vi "Bundle ISD time domain files.vi"(11 "path":path) -> ()   [LabVIEW 2020]
uses:
  <vilib>/Utility/file.llb/Read Delimited Spreadsheet (DBL).vi
  <vilib>/Utility/file.llb/Write Delimited Spreadsheet (string).vi
  <vilib>/Utility/file.llb/Write Delimited Spreadsheet (DBL).vi
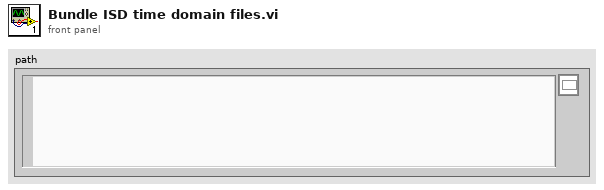
[diagram p1: front panel]
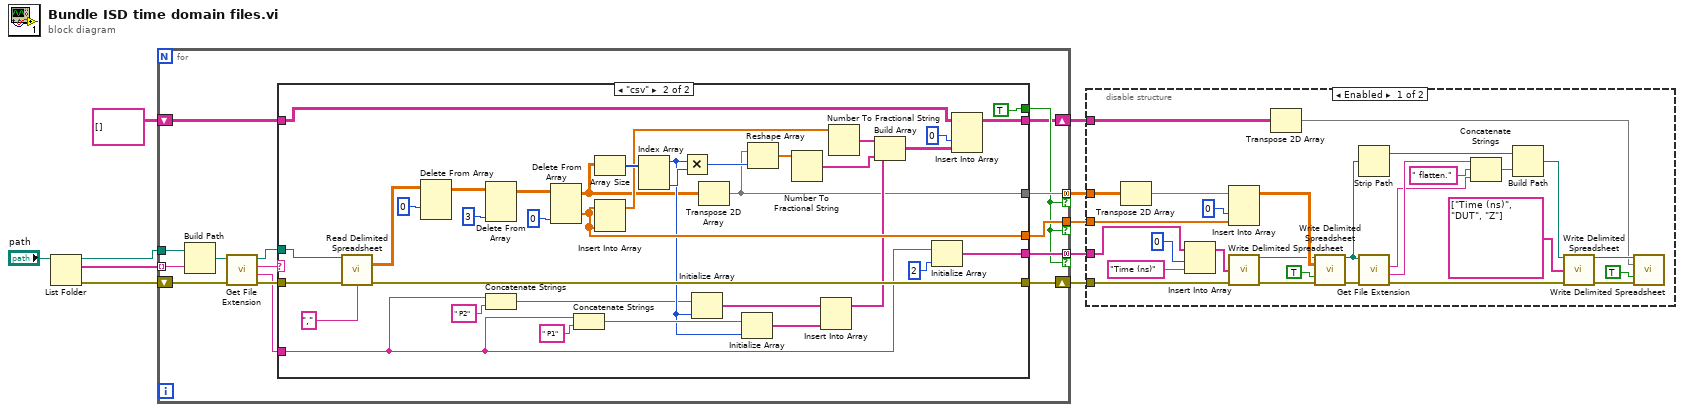
[diagram p0: block diagram]
diagram:
  n1 = List Folder(path="path") -> (path out=w10:path, filenames=w9:string[], error out=w8:errorcluster)  [unwired: 3 in, 1 out]
  n2 = for {
    tunnel: w10 -> [w24]
    tunnel: w9 -> [w23] mode=indexing
    shift-right: [w19] -> w1
    shift-left: w8 -> [w21]
    tunnel: [w17] -> w6 mode=concatenating if=w13
    tunnel: [w16] -> w5 if=w13
    tunnel: [w14] -> w4 mode=concatenating if=w13
    shift-right: [w12] -> w2
    shift-left: string[][] [] -> [w11]
    n3 = Build Path(base path=w24, name or relative path=w23) -> (appended path=w22:path)
    n4 = call <vilib>:"Get File Extension.vi"("error in (no error)"=w21, "file"=w22) -> ("error out"=w20:errorcluster, "filename without extension"=w15:string, "lowercase file extension"=w25:string, "dup file"=w18:path)  [unwired: 5 in, 1 out]
    n5 = case shown="\"csv\"" w25 {
      tunnel: w20 -> [w27 w63]
      tunnel: [w27 w61] -> w19
      tunnel: w18 -> [_ w60]
      tunnel: [_ w28] -> w17
      tunnel: [_ TRUE] -> w13
      tunnel: [_ w40] -> w16
      tunnel: w15 -> [_ w36]
      tunnel: [_ w53] -> w14
      tunnel: [w26 w51] -> w12
      tunnel: w11 -> [w26 w52]
      frame "False", Default {
      }
      frame "csv" {
        n6 = call-poly <vilib>:"Read Delimited Spreadsheet.vi"("file path (dialog if empty)"=w60, "error in (no error)"=w63, "delimiter (\\t)"="," ("delimiter (\\t)")) -> ("all rows"=w57:dbl[][], "error out"=w61:errorcluster)  [unwired: 7 in, 4 out]
        n7 = Delete From Array(array=w57, index (row)=0 ("index")) -> (array with subset deleted=w58:dbl[][])  [unwired: 2 in, 1 out]
        n8 = Delete From Array(array=w58, index (col)=3 ("disabled index (col)")) -> (array with subset deleted=w49:dbl[][])  [unwired: 2 in, 1 out]
        n9 = Concatenate Strings(w36, " P2" ("string")) -> (w30:string)
        n10 = Delete From Array(array=w49, index (col)=0 ("disabled index (col)")) -> (deleted portion=w40:dbl[], array with subset deleted=w29:dbl[][])  [unwired: 2 in]
        n11 = Concatenate Strings(w36, " P1" ("string")) -> (w35:string)
        n12 = Array Size(array=w29) -> (size(s)=w48:i32[])
        n13 = Insert Into Array(array=w40, new element=w40) -> (w39:dbl[])  [unwired: 1 in]
        n14 = Index Array(array=w48) -> (element #1=w34:i32, element #2=w47:i32)  [unwired: 2 in]
        n15 = Multiply(x=w34, y=w47) -> (x*y=w46:i32)
        n16 = Initialize Array(w30, w34) -> (w33:string[])
        n17 = Transpose 2D Array(2D array=w29) -> (transposed array=w28:dbl[][])
        n18 = Initialize Array(w35, w34) -> (w32:string[])
        n19 = Reshape Array(w28, w46) -> (w43:dbl[])
        n20 = Number To Fractional String(number=w43) -> (F-format string=w42:string[])  [unwired: 3 in]
        n21 = Insert Into Array(array=w33, new element=w32) -> (w31:string[])  [unwired: 1 in]
        n22 = Number To Fractional String(number=w39) -> (F-format string=w41:string[])  [unwired: 3 in]
        n23 = Build Array(w41, w31, w42) -> (w45:string[][])
        n24 = Initialize Array(w36, 2 ("dimension size")) -> (w53:string[])
        n25 = Insert Into Array(array=w52, index (col)=0 ("disabled index (col)"), new element=w45) -> (w51:string[][])  [unwired: 1 in]
      }
    }
  }
  n26 = disable-structure shown="Enabled" {
    disable-tunnel: w6 -> [w91 _]
    disable-tunnel: w5 -> [w90 _]
    disable-tunnel: w4 -> [w83 _]
    disable-tunnel: w2 -> [w69 _]
    disable-tunnel: w1 -> [w64 _]
    frame Enabled {
      n27 = Transpose 2D Array(2D array=w91) -> (transposed array=w89:dbl[][])
      n28 = Insert Into Array(array=w83, index=0, new element="Time (ns)" ("new element/subarray")) -> (w67:string[])
      n29 = Insert Into Array(array=w89, index (col)=0 ("disabled index (col)"), new element=w90) -> (w88:dbl[][])  [unwired: 1 in]
      n30 = call-poly <vilib>:"Write Delimited Spreadsheet.vi"("1D data"=w67, "error in (no error)"=w64) -> ("new file path (Not A Path if cancelled)"=w86:path, "error out"=w85:errorcluster)  [unwired: 12 in]
      n31 = Transpose 2D Array(2D array=w69) -> (transposed array=w68:string[][])
      n32 = call-poly <vilib>:"Write Delimited Spreadsheet.vi"("file path (dialog if empty)"=w86, "2D data"=w88, "append to file? (new file:F)"=TRUE, "error in (no error)"=w85) -> ("new file path (Not A Path if cancelled)"=w76:path, "error out"=w77:errorcluster)  [unwired: 10 in]
      n33 = Strip Path(path=w76) -> (stripped path=w72:path)  [unwired: 1 out]
      n34 = call <vilib>:"Get File Extension.vi"("error in (no error)"=w77, "file"=w76) -> ("error out"=w65:errorcluster, "filename without extension"=w75:string, "lowercase file extension"=w73:string)  [unwired: 5 in, 2 out]
      n35 = Concatenate Strings(w75, " flatten." ("string"), w73) -> (w71:string)
      n36 = Build Path(base path=w72, name or relative path=w71) -> (appended path=w70:path)
      n37 = call-poly <vilib>:"Write Delimited Spreadsheet.vi"("file path (dialog if empty)"=w70, "1D data"=string[] ["Time (ns)", "DUT", "Z"], "error in (no error)"=w65) -> ("new file path (Not A Path if cancelled)"=w78:path, "error out"=w79:errorcluster)  [unwired: 11 in]
      n38 = call-poly <vilib>:"Write Delimited Spreadsheet.vi"("file path (dialog if empty)"=w78, "2D data"=w68, "append to file? (new file:F)"=TRUE, "error in (no error)"=w79) -> ()  [unwired: 10 in, 2 out]
    }
    frame Disabled {
    }
  }
